vi "CRYCalc Res Overall yield.vi"(7 "Step Setup VI No":i32, 9 "Statistic Run Number":i32, 11 "Results in":T2 {"Margin" format="%.2f"}) -> (3 "Overall Yield Out":T1[](array[typedef]) {"Z data" items=["dB", "Lin"]; "X data" items=["dB", "Lin"]; "Y data" items=["dB", "Lin"]; "Z dB ref" format="%.1f"; "Z axis" items=["Log", "Lin"]; "X dB ref" format="%.1f"; "X axis" items=["Log", "Lin"]; "Y axis" items=["Log", "Lin"]; "Y dB ref" format="%.1f"; "Curve"."z" format="%.2f"; "Curve"."y" format="%.2f"; "Curve"."x" format="%.2f"})   [LabVIEW 2013]
uses:
  Typedef Control/CRYResult Cluster Array.ctl
  Typedef Control/CRYResult Cluster.ctl
  Typedef Control/CRYData Cluster.ctl
  CRYStatistics Global.vi
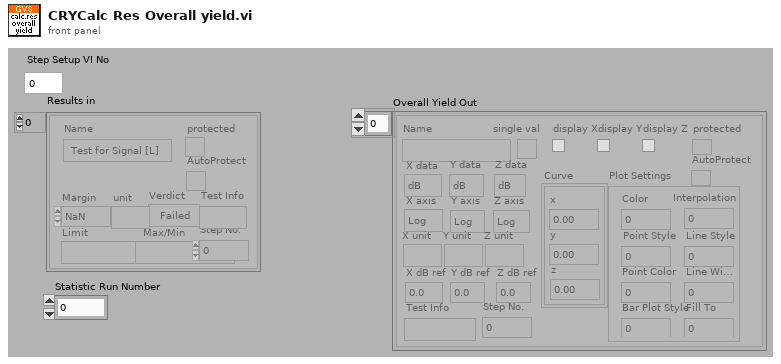
[diagram p1: front panel]
types:
  T1 = typedef "CRYData Cluster.ctl" = cluster{"Name":string, "Curve":cluster{"x":dbl, "y":dbl, "z":dbl}[], "X data":u16, "Y data":u16, "Z data":u16, "X axis":u16, "Y axis":u16, "Z axis":u16, "X unit":string, "Y unit":string, "Z unit":string, "X dB ref":dbl, "Y dB ref":dbl, "Z dB ref":dbl, "single val":bool, "protected":bool, "display X":bool, "display Y":bool, "display Z":bool, "Test Info":string, "Step No.":i32, "Plot Settings":cluster{"Color":u32, "Interpolation":u8, "Point Style":u8, "Line Style":u8, "Point Color":u32, "Line Width":u8, "Bar Plot Style":u8, "Fill To":i16}, "AutoProtect":bool}
  T2 = typedef "CRYResult Cluster Array.ctl" = T3[]
  T3 = typedef "CRYResult Cluster.ctl" = cluster{"Name":string, "Margin":dbl, "unit":string, "Verdict":bool, "Limit":string, "Max/Min":string, "protected":bool, "Step No.":i32, "Test Info":string, "AutoProtect":bool}
  T4 = enum32{"English", "Chinese", "Korean", "Japanese", "Russian", "Chinese traditional"}
  T5 = typedef "CRYData Cluster Array.ctl" = T1[]
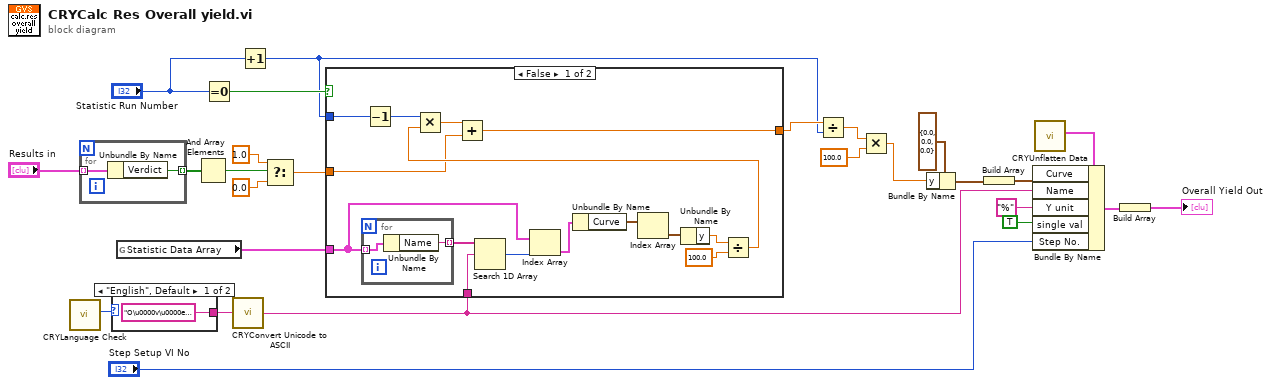
[diagram p0: block diagram]
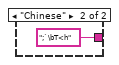
[diagram p3: hidden frame]
diagram:
  n1 = call "CRYLanguage Check.vi"() -> ("Language"=w16:T4)  [unwired: 10 in, 1 out]
  n2 = for {
    tunnel: "Results in" -> [w28] mode=indexing
    tunnel: [w27] -> w14 mode=indexing
    n3 = Unbundle By Name(w28) -> ("Verdict"=w27:bool)
  }
  n4 = case shown="\"English\", Default" w16 {
    tunnel: ["O\u0000v\u0000e\u0000r\u0000a\u0000l\u0000l\u0000 \u0000Y\u0000i\u0000e\u0000l\u0000d\u0000" ("format string") ";`\bT<h" ("format string")] -> w15
    frame "English", Default {
    }
    frame "Chinese" {
    }
  }
  n5 = global read "CRYStatistics Global.vi" "Statistic Data Array"() -> (w12:T5)
  n6 = And Array Elements(Boolean array=w14) -> (logical AND=w8:bool)
  n7 = Equal To 0?(x="Statistic Run Number") -> (x = 0?=w13:bool)
  n8 = call "CRYConvert Unicode to ASCII.vi"("Unicode"=w15) -> ("ASCII"=w11:string)  [unwired: 4 in]
  n9 = Increment(x="Statistic Run Number") -> (x+1=w1:i32)
  n10 = Select(t=1.0, s=w8, f=0.0) -> (s? t:f=w7:dbl)
  n11 = case shown="False" w13 {
    tunnel: w11 -> [w44 _]
    tunnel: w12 -> [w42 _]
    tunnel: w7 -> [w32 w48]
    tunnel: w1 -> [w35 _]
    tunnel: [w31 w48] -> w4
    frame False {
      n12 = for {
        tunnel: w42 -> [w47] mode=indexing
        tunnel: [w46] -> w45 mode=indexing
        n13 = Unbundle By Name(w47) -> ("Name"=w46:string)
      }
      n14 = Decrement(x=w35) -> (x-1=w34:i32)
      n15 = Search 1D Array(1D array=w45, element=w44) -> (index of element=w43:i32)  [unwired: 1 in]
      n16 = Index Array(array=w42, index=w43) -> (element=w41:T1)
      n17 = Unbundle By Name(w41) -> ("Curve"=w40:cluster{"x":dbl, "y":dbl, "z":dbl}[])
      n18 = Index Array(array=w40) -> (element=w39:cluster{"x":dbl, "y":dbl, "z":dbl})  [unwired: 1 in]
      n19 = Unbundle By Name(w39) -> ("y"=w38:dbl)
      n20 = Divide(x=w38, y=100.0) -> (x/y=w36:dbl)
      n21 = Multiply(x=w34, y=w36) -> (x*y=w33:dbl)
      n22 = Add(x=w33, y=w32) -> (x+y=w31:dbl)
    }
    frame True {
    }
  }
  n23 = Divide(x=w4, y=w1) -> (x/y=w5:dbl)
  n24 = Multiply(x=w5, y=100.0) -> (x*y=w2:dbl)
  n25 = Bundle By Name(cluster=cluster{"x":dbl, "y":dbl, "z":dbl} {"x"=0.0, "y"=0.0, "z"=0.0}, "y"=w2) -> (w26:cluster{"x":dbl, "y":dbl, "z":dbl})
  n26 = Build Array(w26) -> (w22:cluster{"x":dbl, "y":dbl, "z":dbl}[])
  n27 = call "CRYUnflatten Data.vi"() -> ("Datum"=w21:T1)  [unwired: 9 in, 2 out]
  n28 = Bundle By Name(cluster=w21, "Curve"=w22, "Name"=w11, "Y unit"="%", "single val"=TRUE, "Step No."="Step Setup VI No") -> (w19:T1)
  n29 = Build Array(w19) -> (→"Overall Yield Out":T1[])
